vi "Update Current Temperature.vi"(8 "error in (no error)":cluster{"状态":bool, "代码":i32, "源":string} caption="错误输入（无错误）", 10 "当前温度":dbl, 11 "冷却器的控制器输入":refnum<class "Cooler Controller.lvclass">) -> (0 "error out":cluster{"状态":bool, "代码":i32, "源":string} caption="错误输出", 3 "冷却器的控制器输出":refnum<class "Cooler Controller.lvclass">)   [LabVIEW 2015, in "Cooler Controller.lvlib" / "Cooler Controller.lvclass"]
doc: "子类必须对该方法进行重写，以便从传感器或仿真源读取系统的当前温度。"
uses:
  Cooler Controller.lvclass
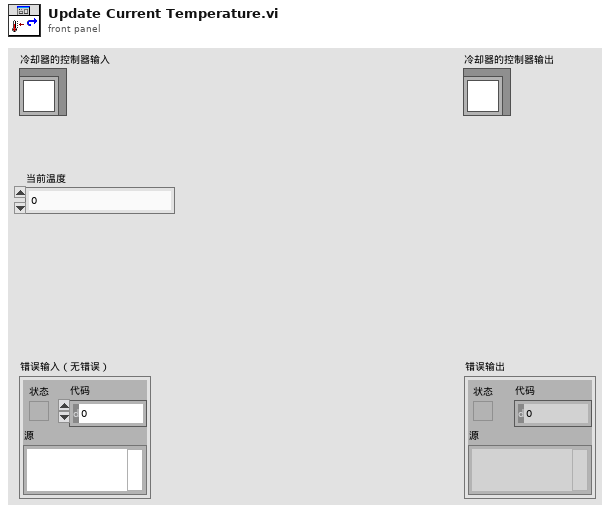
[diagram p1: front panel]
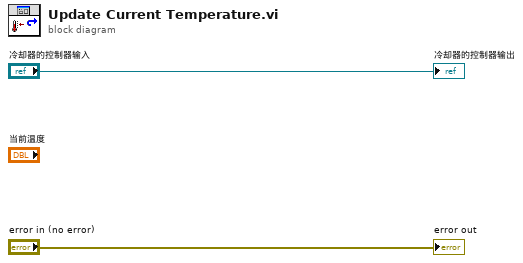
[diagram p0: block diagram]
diagram:
  "error out" <- "error in (no error)"
  "冷却器的控制器输出" <- "冷却器的控制器输入"
